vi "Initialize Parameter Manager.vi"(8 "error in (no error)":errorcluster, 10 "VI Refnum":refnum<vi>, 11 "CD Item Ref":T1=18446744073709551615 format="%.0x") -> (0 "error out":errorcluster, 3 "CD Parameter Manager out":refnum<class "CD Parameter Manager.lvclass">)   [LabVIEW 2016, in "CD Parameter Manager API.lvlib" / "CD Parameter Manager.lvclass"]
uses:
  CD Parameter Manager.lvclass
  <vilib>/NI VeriStand/Custom Device API/Custom Device Item Ref.ctl
  <vilib>/NI VeriStand/Custom Device API/Custom Device API.lvlib
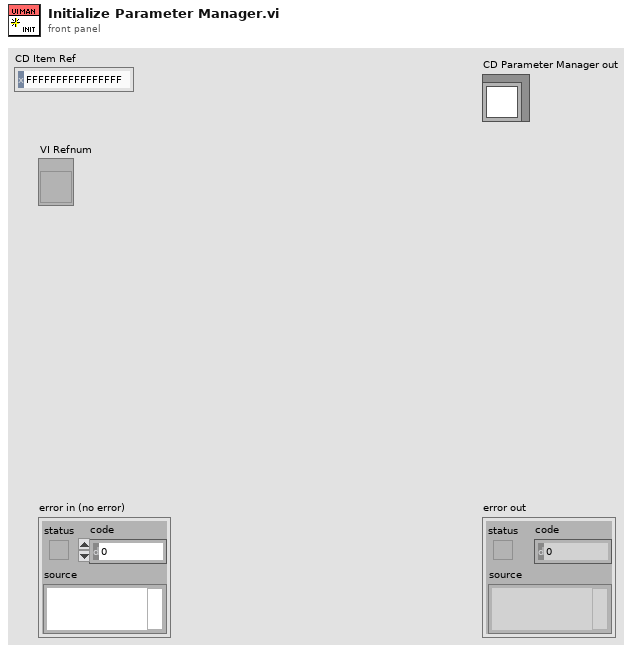
[diagram p1: front panel]
types:
  T1 = typedef "Custom Device API.lvlib/Custom Device Item Ref.ctl" = u64
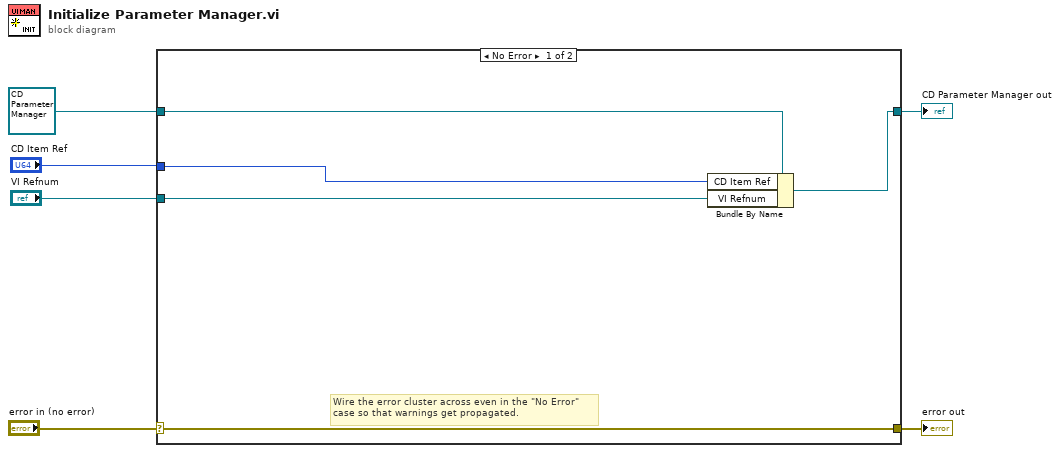
[diagram p0: block diagram]
diagram:
  n1 = case shown="No Error" "error in (no error)" {
    selector: "error in (no error)" -> [w11 w13]
    tunnel: [w11 w13] -> w5
    tunnel: [w8 w12] -> w3
    tunnel: refnum<class "CD Parameter Manager.lvclass"> refnum ("CD Parameter Manager in") -> [w10 w12]
    tunnel: "VI Refnum" -> [w9 _]
    tunnel: "CD Item Ref" -> [w7 _]
    frame No Error {
      # "Wire the error cluster across even in the \"No Error\"\ncase so that warnings get propagated."
      n2 = Bundle By Name(cluster=w10, "CD Item Ref"=w7, "VI Refnum"=w9) -> (w8:refnum<class "CD Parameter Manager.lvclass">)
    }
    frame Error {
    }
  }
  "error out" <- w5
  "CD Parameter Manager out" <- w3
